vi "BLED1112-Advertising  packet parser.vi"(3 "Advertising Data (in)":string[][](array[string])) -> (1 "Advertising Data  (out)":string[][](array[string]))   [LabVIEW 2015]
panel:
  out "porcess no":i32
  # "Advertising  packet parser"
  # "RSSI (power)"
  # "Advertising Package Type"
  # "Friendly name"
  # "MAC Address"
  # "Address Type"
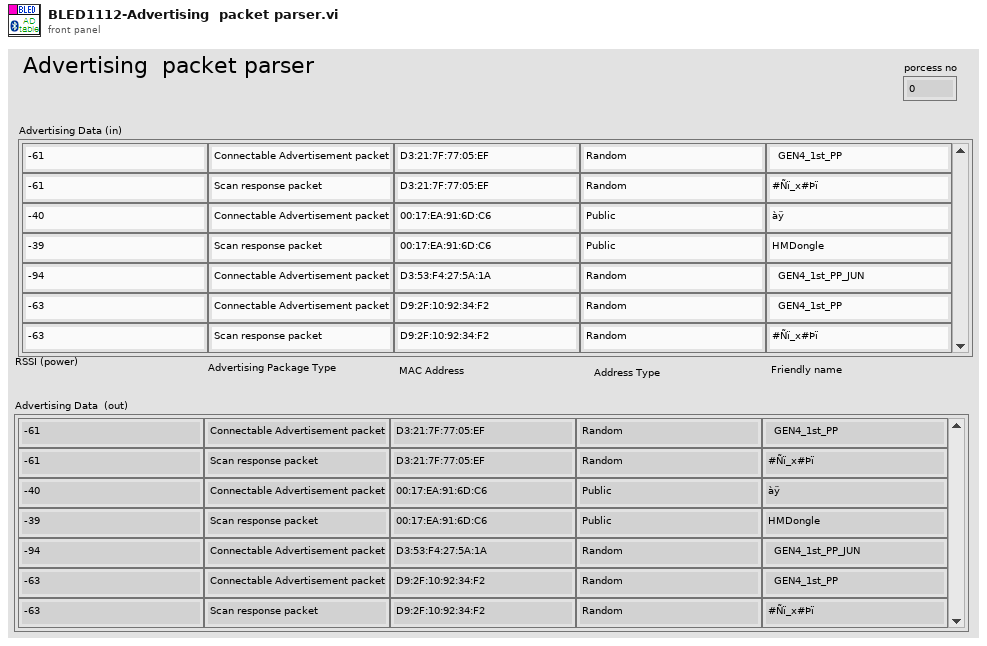
[diagram p1: front panel]
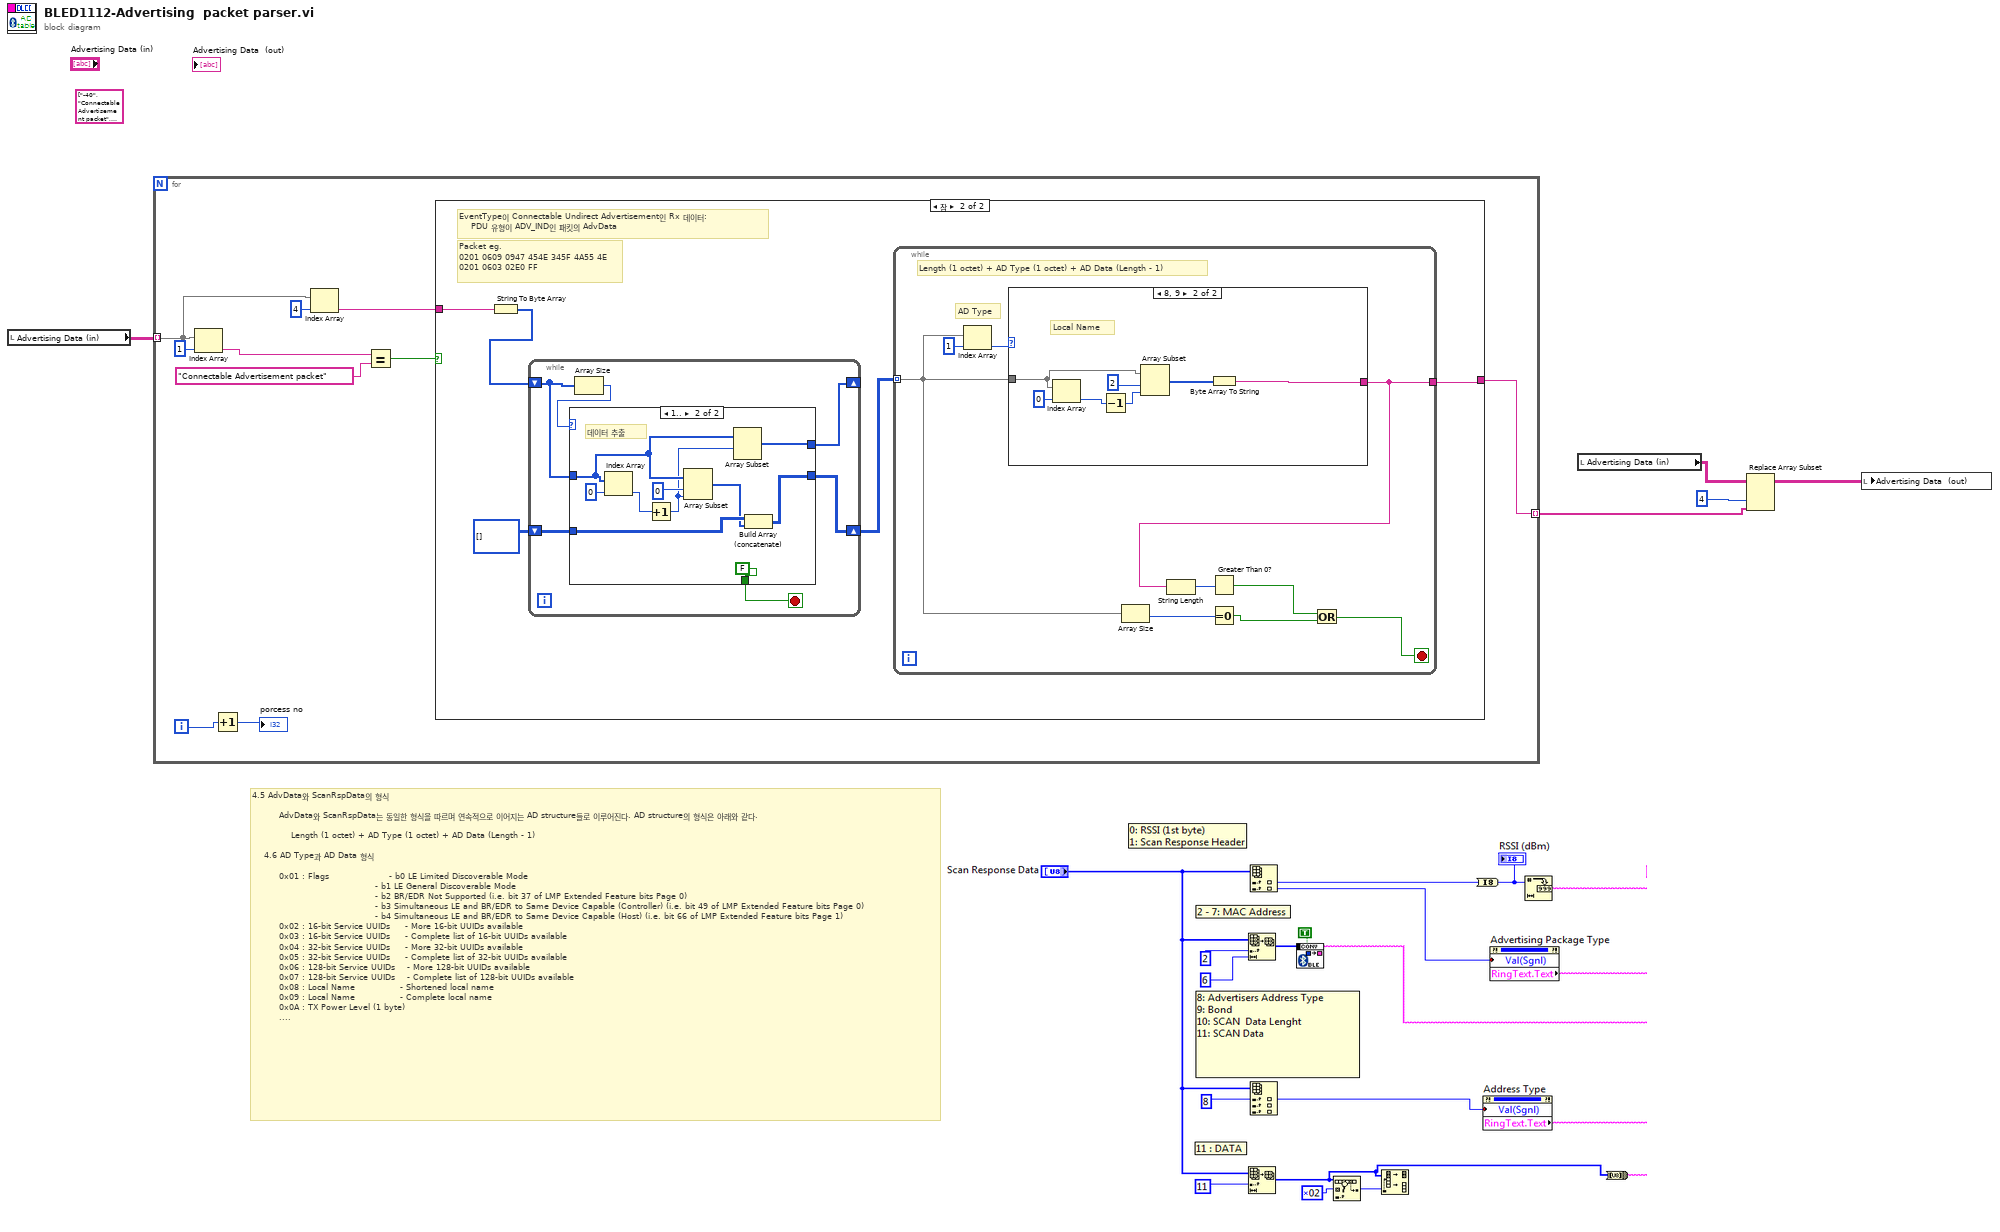
[diagram p0: block diagram]
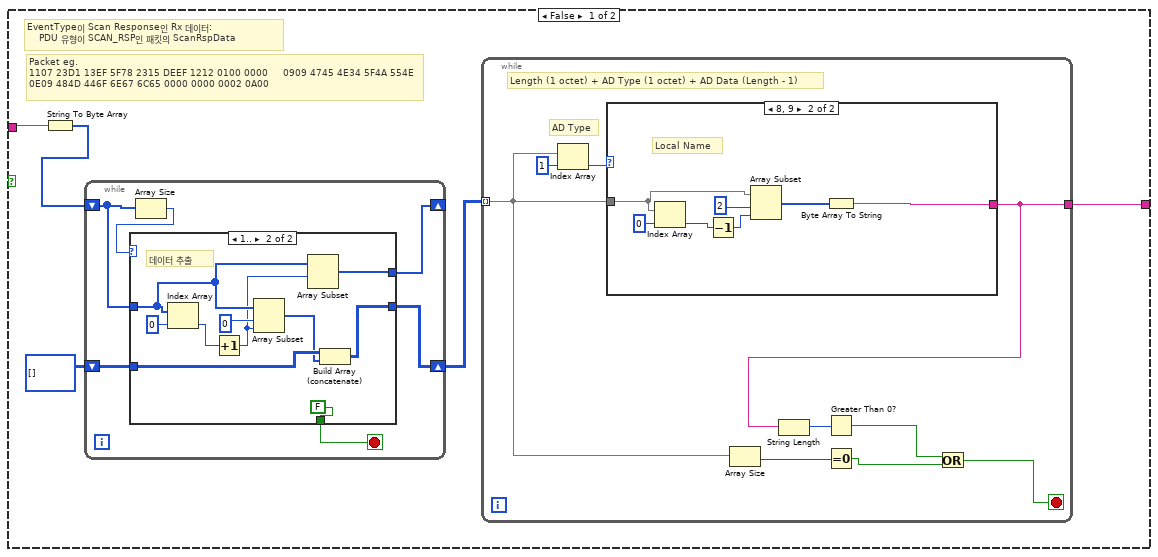
[diagram p2: hidden frame]
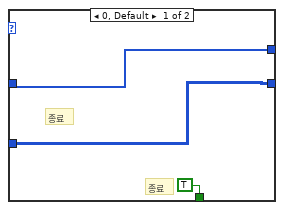
[diagram p4: hidden frame]
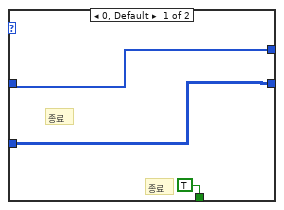
[diagram p6: hidden frame]
diagram:
  (unwired) string[][] [["-40", "Connectable Advertisement packet", "00:17:EA:91:6D:C6", "Public", "\u0002\u0001\u0006\u0003\u0002àÿ"], ["-40", "Scan response packet", "00:17:EA:91:6D:C6", "Public", "\u000e\tHMDongle\u0000\u0000\u0000\u0000\u0000\u0002\n\u0000"], ["-63", "Connectable Advertisement packet", "D3:21:7F:77:05:EF", "Random", "\u0002\u0001\u0006\t\tGEN4_JUN"], ["-63", "Scan response packet", "D3:21:7F:77:05:EF", "Random", "\u0011\u0007#Ñ\u0013ï_x#\u0015Þï\u0012\u0012\u0001\u0000\u0000\u0000\t\tGEN4_JUN"]] ("Devices")
  # "4.5 AdvData와 ScanRspData의 형식\n  \n         AdvData와 ScanRspData는 동일한 형식을 따르며 연속적으로 이어지는 AD structure들로 이루어진다. AD structure의 형식은 아래와 같다.\n\n             Length (1 octet) + AD Type (1 octet) + AD Data (Length - 1)\n           \n    4.6 AD Type과 AD Data 형식\n  \n         0x01 : Flags                    - b0 LE Limited Discoverable Mode\n                                         - b1 LE General Discoverable Mode\n                                         - b2 BR/EDR Not Supported (i.e. bit 37 of LMP Extended Feature bits Page 0)\n                                         - b3 Simultaneous LE and BR/EDR to Same Device Capable (Controller) (i.e. bit 49 of LMP Extended Feature bits Page 0)\n                                         - b4 Simultaneous LE and BR/EDR to Same Device Capable (Host) (i.e. bit 66 of LMP Extended Feature bits Page 1)\n         0x02 : 16-bit Service UUIDs     - More 16-bit UUIDs available\n         0x03 : 16-bit Service UUIDs     - Complete list of 16-bit UUIDs available\n         0x04 : 32-bit Service UUIDs     - More 32-bit UUIDs available\n         0x05 : 32-bit Service UUIDs     - Complete list of 32-bit UUIDs available\n         0x06 : 128-bit Service UUIDs    - More 128-bit UUIDs available\n         0x07 : 128-bit Service UUIDs    - Complete list of 128-bit UUIDs available\n         0x08 : Local Name               - Shortened local name\n         0x09 : Local Name               - Complete local name\n         0x0A : TX Power Level (1 byte)\n         ...."
  n1 = local read "Advertising Data (in)"() -> (w5:string[][])
  n2 = for {
    tunnel: w5 -> [w8] mode=indexing
    tunnel: [w7] -> w4 mode=indexing
    i -> [w14]
    n3 = Index Array(array=w8, index=1 ("인덱스")) -> (element=w11:string)
    n4 = Increment(x=w14) -> (x+1=→"porcess no":i32)
    n5 = Index Array(array=w8, index=4 ("인덱스")) -> (element=w6:string)
    n6 = Equal?(x=w11, y="Connectable Advertisement packet") -> (x = y?=w10:bool)
    n7 = case shown="참" w10 {
      tunnel: w6 -> [w20 w57]
      tunnel: [w16 w56] -> w7
      frame False {
        # "Packet eg.\n1107 23D1 13EF 5F78 2315 DEEF 1212 0100 0000     0909 4745 4E34 5F4A 554E\n0E09 484D 446F 6E67 6C65 0000 0000 0002 0A00"
        # "EventType이 Scan Response인 Rx 데이터:\n    PDU 유형이 SCAN_RSP인 패킷의 ScanRspData"
        n8 = String To Byte Array(string=w20) -> (unsigned byte array=w19:u8[])
        n9 = while {
          shift-right: [w39] -> _
          shift-left: w19 -> [w40]
          shift-right: [w38] -> w17
          shift-left: u8[][] [] -> [w37]
          stop <- w41 stop-if-true
          n10 = Array Size(array=w40) -> (size(s)=w42:i32)
          n11 = case shown="1.." w42 {
            tunnel: [TRUE FALSE] -> w41
            tunnel: w40 -> [w44 w52]
            tunnel: [w43 w49] -> w38
            tunnel: [w44 w48] -> w39
            tunnel: w37 -> [w43 w51]
            frame 0, Default {
              # "종료"
              # "종료"
            }
            frame 1.. {
              # "데이터 추출"
              n12 = Index Array(array=w52, index=0 ("인덱스")) -> (element=w47:u8)
              n13 = Increment(x=w47) -> (x+1=w46:u8)
              n14 = Array Subset(array=w52, index=0 ("인덱스"), length=w46) -> (w50:u8[])
              n15 = Array Subset(array=w52, index=w46) -> (w48:u8[])  [unwired: 1 in]
              n16 = Build Array (concatenate)(w51, w50) -> (w49:u8[][])
            }
          }
        }
        n17 = while {
          tunnel: w17 -> [w27] mode=indexing
          tunnel: [w23] -> w16
          stop <- w24 stop-if-true
          # "Length (1 octet) + AD Type (1 octet) + AD Data (Length - 1)"
          # "AD Type"
          n18 = Index Array(array=w27, index=1 ("인덱스")) -> (element=w28:u8)
          n19 = case shown="8, 9" w28 {
            tunnel: w27 -> [_ w34]
            tunnel: [_ w30] -> w23
            frame 0, Default {
            }
            frame 8, 9 {
              # "Local Name"
              n20 = Index Array(array=w34, index=0 ("인덱스")) -> (element=w32:u8)
              n21 = Decrement(x=w32) -> (x-1=w31:u8)
              n22 = Array Subset(array=w34, index=2 ("인덱스"), length=w31) -> (w33:u8[])
              n23 = Byte Array To String(unsigned byte array=w33) -> (string=w30:string)
            }
          }
          n24 = Array Size(array=w27) -> (size(s)=w26:i32)
          n25 = String Length(string=w23) -> (length=w22:i32)
          n26 = Greater Than 0?(x=w22) -> (x > 0?=w21:bool)
          n27 = Equal To 0?(x=w26) -> (x = 0?=w25:bool)
          n28 = Or(x=w21, y=w25) -> (x .or. y?=w24:bool)
        }
      }
      frame True {
        # "Packet eg.\n0201 0609 0947 454E 345F 4A55 4E\n0201 0603 02E0 FF"
        # "EventType이 Connectable Undirect Advertisement인 Rx 데이터:\n    PDU 유형이 ADV_IND인 패킷의 AdvData"
        n29 = String To Byte Array(string=w57) -> (unsigned byte array=w60:u8[])
        n30 = while {
          shift-right: [w79] -> _
          shift-left: w60 -> [w80]
          shift-right: [w78] -> w58
          shift-left: u8[][] [] -> [w77]
          stop <- w81 stop-if-true
          n31 = Array Size(array=w80) -> (size(s)=w82:i32)
          n32 = case shown="1.." w82 {
            tunnel: [TRUE FALSE] -> w81
            tunnel: w80 -> [w84 w92]
            tunnel: [w83 w89] -> w78
            tunnel: [w84 w88] -> w79
            tunnel: w77 -> [w83 w91]
            frame 0, Default {
              # "종료"
              # "종료"
            }
            frame 1.. {
              # "데이터 추출"
              n33 = Index Array(array=w92, index=0 ("인덱스")) -> (element=w87:u8)
              n34 = Increment(x=w87) -> (x+1=w86:u8)
              n35 = Array Subset(array=w92, index=0 ("인덱스"), length=w86) -> (w90:u8[])
              n36 = Array Subset(array=w92, index=w86) -> (w88:u8[])  [unwired: 1 in]
              n37 = Build Array (concatenate)(w91, w90) -> (w89:u8[][])
            }
          }
        }
        n38 = while {
          tunnel: w58 -> [w67] mode=indexing
          tunnel: [w63] -> w56
          stop <- w64 stop-if-true
          # "Length (1 octet) + AD Type (1 octet) + AD Data (Length - 1)"
          # "AD Type"
          n39 = Index Array(array=w67, index=1 ("인덱스")) -> (element=w68:u8)
          n40 = case shown="8, 9" w68 {
            tunnel: w67 -> [_ w74]
            tunnel: [_ w70] -> w63
            frame 0, Default {
            }
            frame 8, 9 {
              # "Local Name"
              n41 = Index Array(array=w74, index=0 ("인덱스")) -> (element=w72:u8)
              n42 = Decrement(x=w72) -> (x-1=w71:u8)
              n43 = Array Subset(array=w74, index=2 ("인덱스"), length=w71) -> (w73:u8[])
              n44 = Byte Array To String(unsigned byte array=w73) -> (string=w70:string)
            }
          }
          n45 = Array Size(array=w67) -> (size(s)=w66:i32)
          n46 = String Length(string=w63) -> (length=w62:i32)
          n47 = Greater Than 0?(x=w62) -> (x > 0?=w61:bool)
          n48 = Equal To 0?(x=w66) -> (x = 0?=w65:bool)
          n49 = Or(x=w61, y=w65) -> (x .or. y?=w64:bool)
        }
      }
    }
  }
  n50 = local read "Advertising Data (in)"() -> (w1:string[][])
  n51 = Replace Array Subset(array=w1, new element=w4, index (col)=4 ("비활성화된 인덱스 (열)")) -> (w3:string[][])  [unwired: 1 in]
  n52 = local write "Advertising Data  (out)"(w3) -> ()
